vi "FitnessOnTestData.vi"(8 "Test Data":T1=enum."Test Data", 9 "Training Data":T1, 10 "Phenotype":i32[](array[numeric]), 11 "BandGlobalOpt.lvclass":refnum<class "OptFreqBandsSearch.lvclass">) -> (1 "Fitness":dbl)   [LabVIEW 2016, in "Optimal Frequency Bands Search.lvlib" / "GeneticAlgorithm.lvlib"]
doc: "Процедура оценки точности классификации. Для оценки точности классификации классификатор на основе многослойного персептрона обучается на обучающих данных, тестируется - на тестовых."
uses:
  GeneticAlgorithm.lvlib
  _vlib/OptFreqBandsSearch.lvclass
  _vlib/OFBS_DataTypes.ctl
  Optimal Frequency Bands Search.lvlib
panel:
  # "This VI is a part of BCI Design library, http://www.ru-bci.org \nCopyright © 2020, Sotnikov Peter, All rights reserved. License: CC BY-NC 4.0"
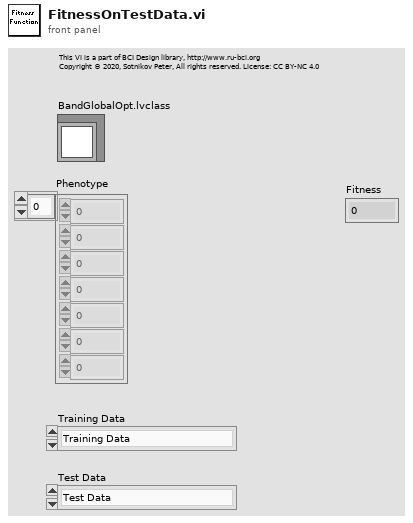
[diagram p1: front panel]
types:
  T1 = typedef "Optimal Frequency Bands Search.lvlib/OFBS_DataTypes.ctl" = enum16{"Training Data", "Test Data", "Training Data (cross-check)", "Test Data (cross-check)"}
  T2 = typedef "Optimal Frequency Bands Search.lvlib/OFBS_ClassifierTypes.ctl" = enum16{"Multilayer perceptron", "k NN Classifier", "SVM Committee", "Mahalanobis distance", "SVM Classifier"}
  T3 = typedef "NILabs_MLT.lvlib/ml_BP_Project.ctl" = cluster{"Training Data":T4, "Normalize Info":T5, "3-layer NN":T6, "Ternimal Condition":T7}
  T4 = typedef "NILabs_MLT.lvlib/ml_BP_Data.ctl" = cluster{"dim in":i32, "dim out":i32, "# samples":i32, "Input":dbl[][], "Output":dbl[][]}
  T5 = typedef "NILabs_MLT.lvlib/ml_BP_Normalize Data.ctl" = cluster{"input min":dbl[], "input max":dbl[], "output min":dbl[], "output max":dbl[]}
  T6 = typedef "NILabs_MLT.lvlib/ml_BP_3layer Feedforward.ctl" = cluster{"# input neuron ":i32, "# hidden neuron":i32, "# output neuron":i32, "Weight (I->H)":dbl[][], "Weight (H->O)":dbl[][], "Output":dbl[][], "Hidden Out":dbl[][], "Derivation Output":dbl[][], "Derivation Hidden":dbl[][], "dw (I->H)":dbl[][], "dw (H->O)":dbl[][]}
  T7 = typedef "NILabs_MLT.lvlib/ml_BP_Terminal Condition.ctl" = cluster{"min MSE":dbl, "min delta MSE":dbl, "min step length":dbl, "max iteration":dbl}
  T8 = typedef "IMAQ Classifier Session.ctl" = refnum<k1>
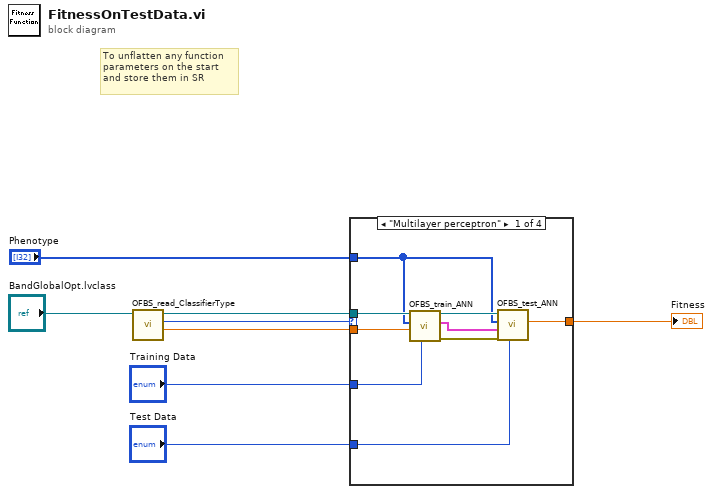
[diagram p0: block diagram]
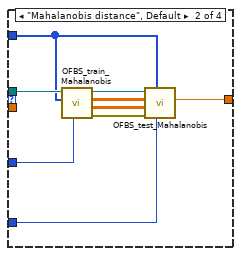
[diagram p2: hidden frame]
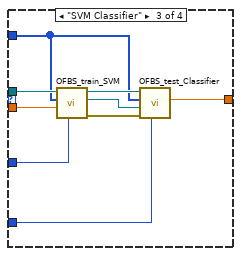
[diagram p3: hidden frame]
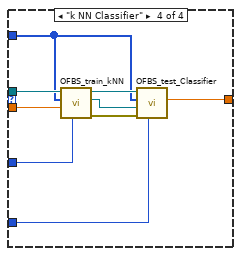
[diagram p4: hidden frame]
diagram:
  # "To unflatten any function\nparameters on the start\nand store them in SR"
  n1 = call-dynamic "OFBS_read_ClassifierType.vi"("OptFreqBandsSearch in"="BandGlobalOpt.lvclass") -> ("Classifier Metaparameter"=w1:dbl, "ClassifierType"=w5:T2, "OptFreqBandsSearch out"=w6:refnum<class "OptFreqBandsSearch.lvclass">)  [unwired: 7 in, 1 out]
  n2 = case shown="\"Multilayer perceptron\"" w5 {
    tunnel: [w17 w22 w32 w41] -> w2
    tunnel: w6 -> [w13 w21 w31 w40]
    tunnel: "Phenotype" -> [w12 w18 w28 w39]
    tunnel: "Training Data" -> [w10 w20 w30 w38]
    tunnel: "Test Data" -> [w11 w19 w29 w37]
    tunnel: w1 -> [w9 _ w27 w36]
    frame "Multilayer perceptron" {
      n3 = call "OFBS_train_ANN.vi"("Train Data"=w10, "# of hidden neurons"=w9, "Parameters"=w12, "OFBS class in"=w13) -> ("error out"=w14:errorcluster, "ANN out"=w15:T3, "OFBS class out"=w16:refnum<class "OptFreqBandsSearch.lvclass">)  [unwired: 4 in, 1 out]
      n4 = call "OFBS_test_ANN.vi"("Test Data"=w11, "error in (no error)"=w14, "ANN in"=w15, "Parameters"=w12, "OFBS class in"=w16) -> ("Accuracy"=w17:dbl)  [unwired: 3 in, 3 out]
    }
    frame "Mahalanobis distance", Default {
      n5 = call "OFBS_train_Mahalanobis.vi"("Train Data"=w20, "Parameters"=w18, "OFBS class in"=w21) -> ("error out"=w23:errorcluster, "Mean vectors"=w24:dbl[][], "Covariance matricies (inversed)"=w25:dbl[][][], "OFBS class out"=w26:refnum<class "OptFreqBandsSearch.lvclass">)  [unwired: 5 in]
      n6 = call "OFBS_test_Mahalanobis.vi"("Test Data"=w19, "Parameters"=w18, "error in (no error)"=w23, "Mean vectors"=w24, "Covariance matricies (inversed)"=w25, "OFBS class in"=w26) -> ("Accuracy"=w22:dbl)  [unwired: 2 in, 3 out]
    }
    frame "SVM Classifier" {
      n7 = call "OFBS_train_SVM.vi"("Train Data"=w30, "Nu"=w27, "Parameters"=w28, "OFBS class in"=w31) -> ("error out"=w33:errorcluster, "Classifier Session (out)"=w34:T8, "OFBS class out"=w35:refnum<class "OptFreqBandsSearch.lvclass">)  [unwired: 4 in, 1 out]
      n8 = call "OFBS_test_Classifier.vi"("Test Data"=w29, "error in (no error)"=w33, "Classifier Session"=w34, "Parameters"=w28, "OFBS class in"=w35) -> ("Accuracy"=w32:dbl)  [unwired: 3 in, 3 out]
    }
    frame "k NN Classifier" {
      n9 = call "OFBS_train_kNN.vi"("Train Data"=w38, "k"=w36, "Parameters"=w39, "OFBS class in"=w40) -> ("error out"=w43:errorcluster, "Classifier Session (out)"=w42:T8, "OFBS class out"=w44:refnum<class "OptFreqBandsSearch.lvclass">)  [unwired: 4 in, 1 out]
      n10 = call "OFBS_test_Classifier.vi"("Test Data"=w37, "error in (no error)"=w43, "Classifier Session"=w42, "Parameters"=w39, "OFBS class in"=w44) -> ("Accuracy"=w41:dbl)  [unwired: 3 in, 3 out]
    }
  }
  "Fitness" <- w2
